vi "Convert Direction Parameters.vi"(9 "Flip Vertical":bool, 10 "Flip Horizontal":bool, 11 "Display Direction":T1) -> (2 "Top To Bottom":bool, 3 "Left To Right":bool, 5 "Flip Axis":bool)   [LabVIEW 2020, in "RPI.SenseHat.Display.lvlib"]
uses:
  RPI.SenseHat.Display.lvlib
  TypeDefs/Display Direction.ctl
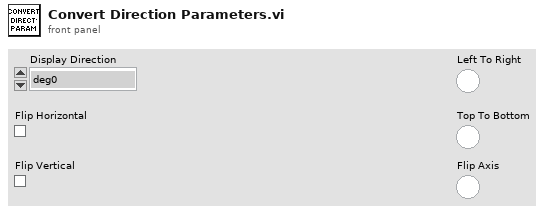
[diagram p1: front panel]
types:
  T1 = typedef "RPI.SenseHat.Display.lvlib/Display Direction.ctl" = enum16{"deg0", "deg90", "deg180", "deg270"}
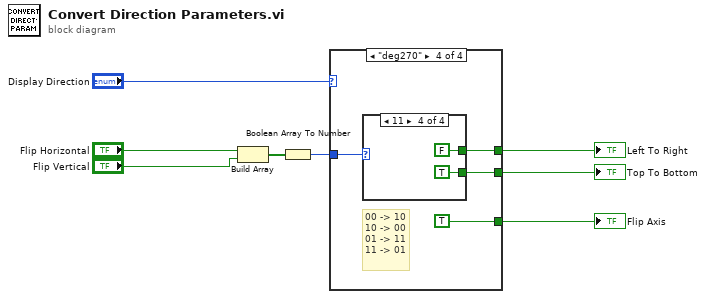
[diagram p0: block diagram]
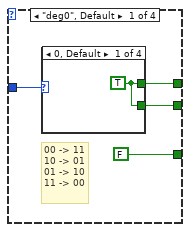
[diagram p2: hidden frame]
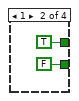
[diagram p3: hidden frame]
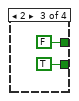
[diagram p4: hidden frame]
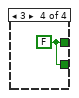
[diagram p5: hidden frame]
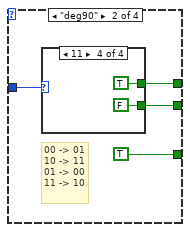
[diagram p6: hidden frame]
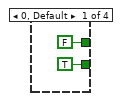
[diagram p7: hidden frame]
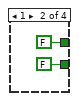
[diagram p8: hidden frame]
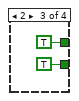
[diagram p9: hidden frame]
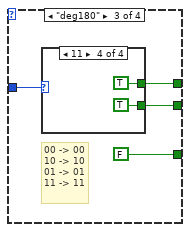
[diagram p10: hidden frame]
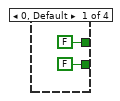
[diagram p11: hidden frame]
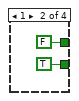
[diagram p12: hidden frame]
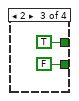
[diagram p13: hidden frame]
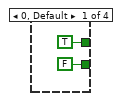
[diagram p14: hidden frame]
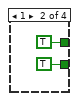
[diagram p15: hidden frame]
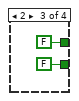
[diagram p16: hidden frame]
diagram:
  n1 = Build Array("Flip Horizontal", "Flip Vertical") -> (w2:bool[])
  n2 = Boolean Array To Number(Boolean array=w2) -> (number=w1:u32)
  n3 = case shown="\"deg270\"" "Display Direction" {
    tunnel: w1 -> [w12 w22 w34 w46]
    tunnel: [w11 w21 w33 w45] -> w5
    tunnel: [w10 w20 w32 w44] -> w4
    tunnel: [FALSE TRUE FALSE TRUE] -> w3
    frame "deg0", Default {
      # "00 -> 11\n10 -> 01\n01 -> 10\n11 -> 00"
      n4 = case shown="0, Default" w12 {
        tunnel: [w13 TRUE FALSE w18] -> w11
        tunnel: [w13 FALSE TRUE w18] -> w10
        frame 0, Default {
          w13 = TRUE
        }
        frame 1 {
        }
        frame 2 {
        }
        frame 3 {
          w18 = FALSE
        }
      }
    }
    frame "deg90" {
      # "00 -> 01\n10 -> 11\n01 -> 00\n11 -> 10"
      n5 = case shown="11" w22 {
        tunnel: [FALSE FALSE TRUE TRUE] -> w21
        tunnel: [TRUE FALSE TRUE FALSE] -> w20
        frame 0, Default {
        }
        frame 1 {
        }
        frame 2 {
        }
        frame 3 {
        }
      }
    }
    frame "deg180" {
      # "00 -> 00\n10 -> 10\n01 -> 01\n11 -> 11"
      n6 = case shown="11" w34 {
        tunnel: [FALSE FALSE TRUE TRUE] -> w33
        tunnel: [FALSE TRUE FALSE TRUE] -> w32
        frame 0, Default {
        }
        frame 1 {
        }
        frame 2 {
        }
        frame 3 {
        }
      }
    }
    frame "deg270" {
      # "00 -> 10\n10 -> 00\n01 -> 11\n11 -> 01"
      n7 = case shown="11" w46 {
        tunnel: [TRUE TRUE FALSE FALSE] -> w45
        tunnel: [FALSE TRUE FALSE TRUE] -> w44
        frame 0, Default {
        }
        frame 1 {
        }
        frame 2 {
        }
        frame 3 {
        }
      }
    }
  }
  "Left To Right" <- w5
  "Top To Bottom" <- w4
  "Flip Axis" <- w3
